vi "Read Open Close Logic.vi"(8 "error in (no error)":errorcluster, 11 "Form Server Configuration in":refnum<class "Form Server Configuration.lvclass">) -> (0 "error out":errorcluster, 2 "Form Server Interfaces.lvlib:Open Close Logic.lvclass":refnum<class "Open Close Logic.lvclass">, 3 "Form Server Configuration out":refnum<class "Form Server Configuration.lvclass">)   [LabVIEW 2020, in "Form Server Configuration.lvlib" / "Form Server Configuration.lvclass"]
uses:
  Form Server Configuration.lvclass
  Autoclose manager/Open Close Logic.lvclass
  Form Server Configuration.lvclass/Form Server Configuration.ctl
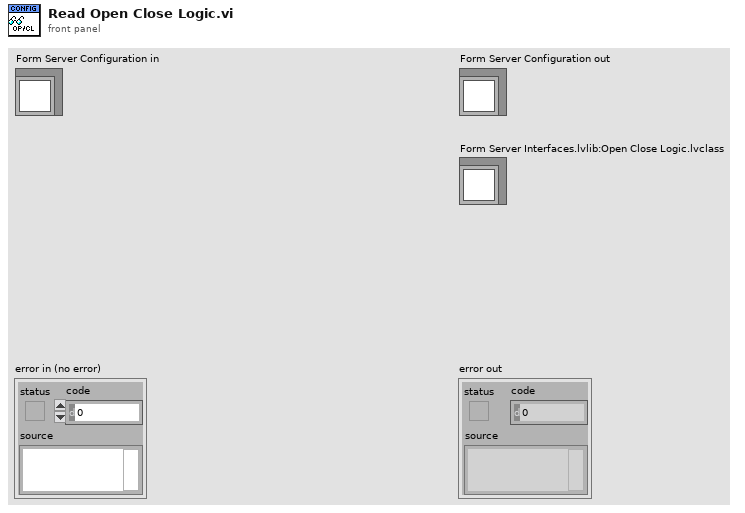
[diagram p1: front panel]
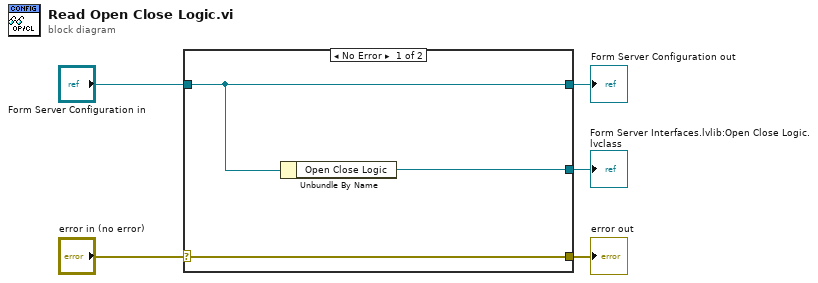
[diagram p0: block diagram]
diagram:
  n1 = case shown="No Error" "error in (no error)" {
    selector: "error in (no error)" -> [w8 w9]
    tunnel: [w8 w9] -> w4
    tunnel: [w7 w10] -> w2
    tunnel: "Form Server Configuration in" -> [w7 w10]
    tunnel: [w6 _] -> w1
    frame No Error {
      n2 = Unbundle By Name(w7) -> ("Open Close Logic"=w6:refnum<class "Open Close Logic.lvclass">)
    }
    frame Error {
    }
  }
  "error out" <- w4
  "Form Server Configuration out" <- w2
  "Form Server Interfaces.lvlib:Open Close Logic.lvclass" <- w1
